vi "Measurement Logic.vi"(8 "error in":errorcluster, 9 "measurement configuration":T2 {"PAYLOAD" format="%x"; "TYPE" items=["CAN Data"=0, "CAN Remote"=1, "CAN Bus Error"=2, "CAN 2.0 Data"=8, "CAN FD Data"=16, "CAN FD+BRS Data"=24, "J1939 Data"=192, "Delay"=224, "Log Trigger"=225, "Start Trigger"=226]; "IDENTIFIER" format="%x"; "Baudrate" format="%x"; "FD Baudrate" format="%x"}, 10 "measure call context in":refnum<class "Measure Call Context.lvclass">) -> (0 "error out":errorcluster, 1 "measurement results":T1, 2 "measure call context out":refnum<class "Measure Call Context.lvclass">)   [LabVIEW 2025, in "CAN-LIN Frame Generator.lvclass"]
doc: "Contains the core logic for executing the measurement."
uses:
  CAN-LIN Frame Generator.lvclass
  <vilib>/Plug-In SDKs/Measurements/Measure Call Context/Measure Call Context.lvclass
  Measurement Configuration.ctl
  Measurement Results.ctl
  <vilib>/xnet/xnet.llb/XNET Frame CAN.ctl
  <vilib>/xnet/xnet.llb/XNET Frame Type CAN.ctl
  <vilib>/xnet/xnet.llb/XNET Create Session (Frame Output Stream).vi
  <vilib>/xnet/xnet.llb/XNET Write (Frame CAN).vi
  <vilib>/xnet/xnet.llb/XNET Wait (Transmit Complete).vi
  <extravilib>/ChannelInstances/Event Messenger-bool/Instantiate.vi
  <resource>/objmgr/xnet.rc
  session-management/xnetCAN/Session Management xnetCAN.lvlib
  <vilib>/Plug-In SDKs/Clients/Session Management V1/Session Reservation/Session Reservation.lvclass
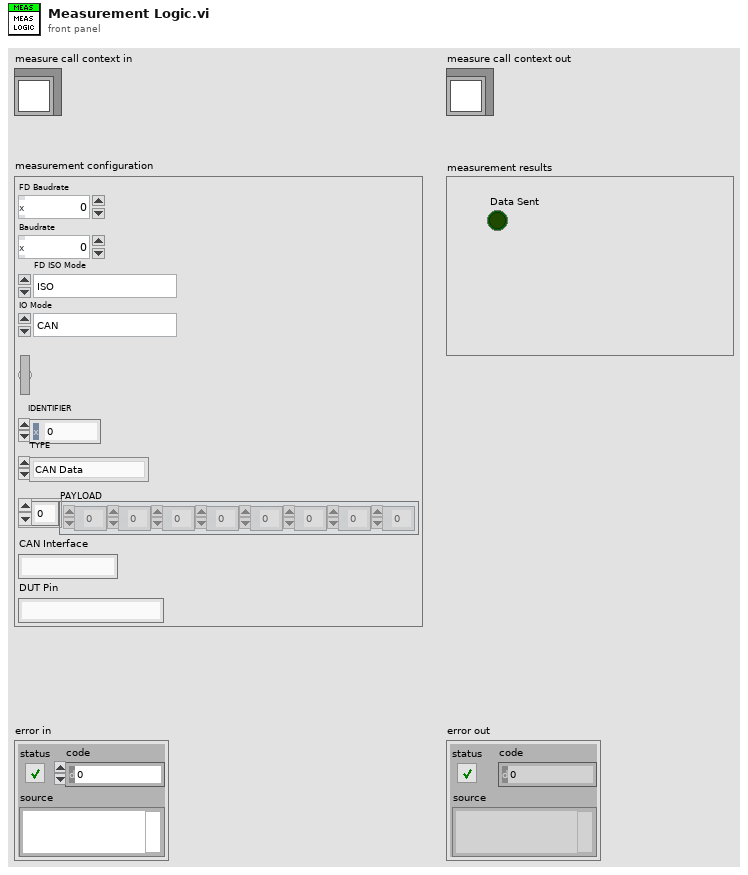
[diagram p1: front panel]
types:
  T1 = typedef "CAN-LIN Frame Generator.lvclass/Measurement Results.ctl" = cluster{"Data Sent":bool}
  T2 = typedef "CAN-LIN Frame Generator.lvclass/Measurement Configuration.ctl" = cluster{"FD Baudrate":u32, "Baudrate":u32, "FD ISO Mode":enum32{"ISO", "Legacy ISO", "Non-ISO"}, "IO Mode":enum32{"CAN", "CAN FD", "CAN FD + BRS"}, "Termination CAN":bool, "IDENTIFIER":u32, "TYPE":u32, "PAYLOAD":u32[], "CAN Interface":string, "DUT Pin":string}
  T3 = typedef "XNET Frame CAN.ctl" = cluster{"timestamp":timestamp, "payload":u8[], "identifier":u32, "type":T4, "extended?":bool, "echo?":bool}
  T4 = typedef "XNET Frame Type CAN.ctl" = u8
  T5 = typedef "Event Messenger-bool.lvlib/))Channel.ctl" = refnum<queue>
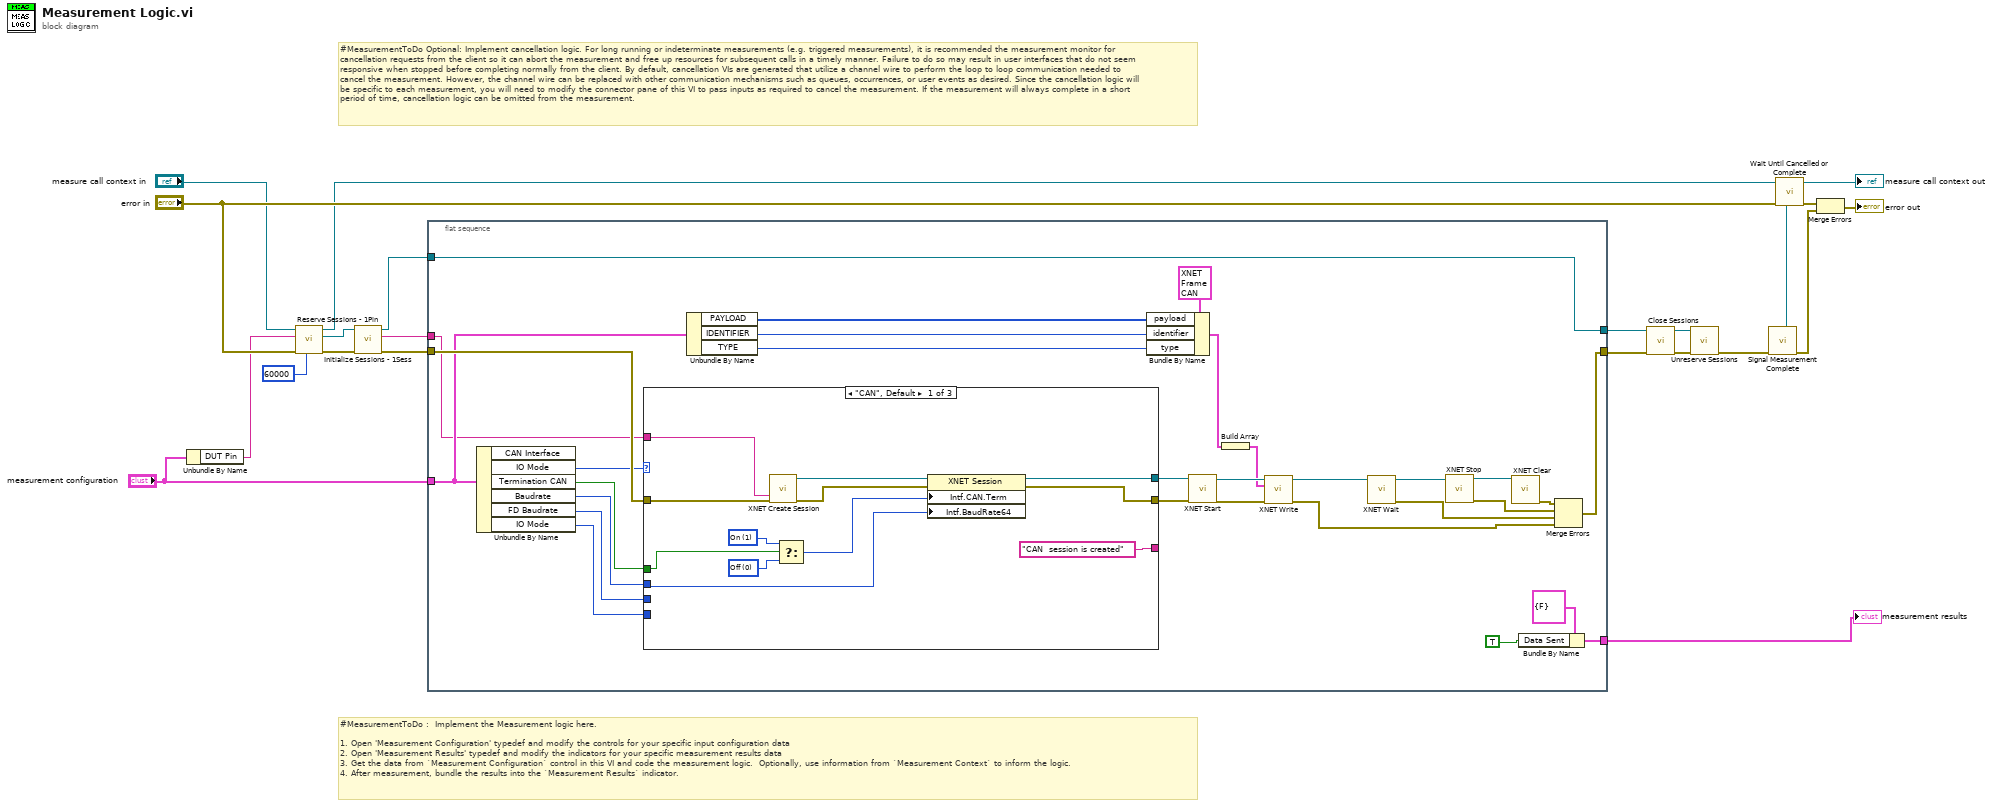
[diagram p0: block diagram]
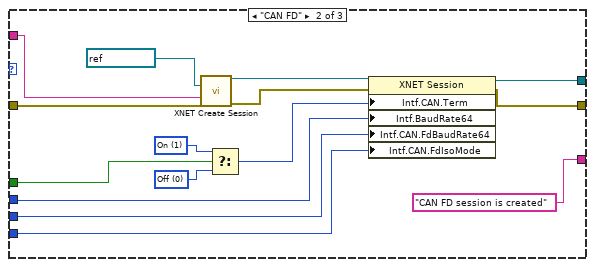
[diagram p2: hidden frame]
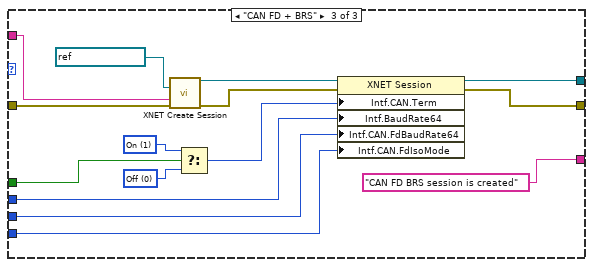
[diagram p3: hidden frame]
diagram:
  # "#MeasurementToDo Optional: Implement cancellation logic. For long running or indeterminate measurements (e.g. triggered measurements), it is recommended the measurement monitor for cancellation requests from the client so it can abort the measurement and free up resources for subsequent calls in a timely manner. Failure to do so may result in user interfaces that do not seem responsive when stopped before completing normally from the client. By default, cancellation VIs are generated that utilize a channel wire to perform the loop to loop communication needed to cancel the measurement. However, the channel wire can be replaced with other communication mechanisms such as queues, occurrences, or user events as desired. Since the cancellation logic will be specific to each measurement, you will need to modify the connector pane of this VI to pass inputs as required to cancel the measurement. If the measurement will always complete in a short period of time, cancellation logic can be omitted from the measurement."
  # "#MeasurementToDo :  Implement the Measurement logic here.\n\n1. Open 'Measurement Configuration' typedef and modify the controls for your specific input configuration data\n2. Open 'Measurement Results' typedef and modify the indicators for your specific measurement results data\n3. Get the data from `Measurement Configuration` control in this VI and code the measurement logic.  Optionally, use information from `Measurement Context` to inform the logic.\n4. After measurement, bundle the results into the `Measurement Results` indicator."
  n1 = Unbundle By Name("measurement configuration") -> ("DUT Pin"=w1:string)
  n2 = call <vilib>:"Reserve Sessions - 1Pin.vi"("timeout (ms)"=60000 ("timeout in milliseconds"), "error in"="error in", "pin or relay name"=w1, "measurement context in"="measure call context in") -> ("error out"=w11:errorcluster, "session reservation out"=w14:refnum<class "Session Reservation.lvclass">, "measurement context out"=w12:refnum<class "Measure Call Context.lvclass">)  [unwired: 5 in]
  n3 = call "Initialize Sessions - 1Sess.vi"("error in"=w11, "session reservation in"=w14) -> ("error out"=w10:errorcluster, "session"=w3:string, "session reservation out"=w4:refnum<class "Session Reservation.lvclass">)  [unwired: 6 in, 1 out]
  n4 = flat-sequence {
    tunnel: "measurement configuration" -> [w28]
    tunnel: w10 -> [w52]
    tunnel: [w30] -> w7
    tunnel: [w42] -> w17
    tunnel: [w24] -> w5
    tunnel: w4 -> [w24]
    tunnel: w3 -> [w23]
    frame #0 {
      n5 = Unbundle By Name(w28) -> ("IO Mode"=w40:enum32{"CAN", "CAN FD", "CAN FD + BRS"}, "Termination CAN"=w51:bool, "Baudrate"=w50:u32, "FD Baudrate"=w49:u32, "IO Mode"=w48:enum32{"CAN", "CAN FD", "CAN FD + BRS"})  [unwired: 1 out]
      n6 = case shown="\"CAN\", Default" w40 {
        tunnel: [w59 w69 w88] -> w47
        tunnel: w52 -> [w58 w73 w83]
        tunnel: [w57 w68 w82] -> w46
        tunnel: w51 -> [w56 w72 w87]
        tunnel: w50 -> [w55 w71 w86]
        tunnel: w49 -> [_ w67 w85]
        tunnel: w48 -> [_ w70 w84]
        tunnel: ["CAN  session is created" ("message") "CAN FD session is created" ("message") "CAN FD BRS session is created" ("message")] -> _
        tunnel: w23 -> [w53 w65 w80]
        frame "CAN", Default {
          w62 = u32 1 items=["Off", "On"] ("Interface:CAN:Termination")
          w61 = u32 0 items=["Off", "On"] ("Interface:CAN:Termination")
          n7 = call-poly <vilib>:"XNET Create Session.vi"("interface"=w53, "error in (no error)"=w58) -> ("session out"=w64:refnum<k21>, "error out"=w63:errorcluster)  [unwired: 12 in]
          n8 = Select(t=w62, s=w56, f=w61) -> (s? t:f=w60:u32)
          n9 = property class="XNET Session"(reference=w64, error in=w63, "Intf.CAN.Term"=w60, "Intf.BaudRate64"=w55) -> (reference out=w59:refnum<k21>, error out=w57:errorcluster)
        }
        frame "CAN FD" {
          w76 = u32 1 items=["Off", "On"] ("Interface:CAN:Termination")
          w75 = u32 0 items=["Off", "On"] ("Interface:CAN:Termination")
          n10 = call-poly <vilib>:"XNET Create Session.vi"("cluster (:memory:)"=refnum<k21> ":can_fd:", "interface"=w65, "error in (no error)"=w73) -> ("session out"=w78:refnum<k21>, "error out"=w77:errorcluster)  [unwired: 11 in]
          n11 = Select(t=w76, s=w72, f=w75) -> (s? t:f=w74:u32)
          n12 = property class="XNET Session"(reference=w78, error in=w77, "Intf.CAN.Term"=w74, "Intf.BaudRate64"=w71, "Intf.CAN.FdBaudRate64"=w67, "Intf.CAN.FdIsoMode"=w70) -> (reference out=w69:refnum<k21>, error out=w68:errorcluster)
        }
        frame "CAN FD + BRS" {
          w91 = u32 1 items=["Off", "On"] ("Interface:CAN:Termination")
          w90 = u32 0 items=["Off", "On"] ("Interface:CAN:Termination")
          n13 = call-poly <vilib>:"XNET Create Session.vi"("cluster (:memory:)"=refnum<k21> ":can_fd_brs:", "interface"=w80, "error in (no error)"=w83) -> ("session out"=w93:refnum<k21>, "error out"=w92:errorcluster)  [unwired: 11 in]
          n14 = Select(t=w91, s=w87, f=w90) -> (s? t:f=w89:u32)
          n15 = property class="XNET Session"(reference=w93, error in=w92, "Intf.CAN.Term"=w89, "Intf.BaudRate64"=w86, "Intf.CAN.FdBaudRate64"=w85, "Intf.CAN.FdIsoMode"=w84) -> (reference out=w88:refnum<k21>, error out=w82:errorcluster)
        }
      }
      n16 = Unbundle By Name(w28) -> ("PAYLOAD"=w27:u32[], "IDENTIFIER"=w26:u32, "TYPE"=w25:u32)
      n17 = Bundle By Name(cluster=T3 {"timestamp"=timestamp(0 s since 1904-01-01), "payload"=[1, 2, 3, 4, 5, 6, 7, 8], "identifier"=2, "type"=0, "extended?"=FALSE, "echo?"=FALSE} ("CAN frame"), "payload"=w27, "identifier"=w26, "type"=w25) -> (w38:T3)
      n18 = call <vilib>:"XNET Start.vi"("session in"=w47, "error in (no error)"=w46) -> ("session out"=w45:refnum<k21>, "error out"=w44:errorcluster)  [unwired: 12 in]
      n19 = Build Array(w38) -> (w37:T3[])
      n20 = call-poly <vilib>:"XNET Write.vi"("session in"=w45, "data"=w37, "error in (no error)"=w44) -> ("session out"=w36:refnum<k21>, "error out"=w29:errorcluster)  [unwired: 11 out]
      n21 = call-poly <vilib>:"XNET Wait.vi"("session in"=w36) -> ("session out"=w35:refnum<k21>, "error out"=w31:errorcluster)  [unwired: 13 in]
      n22 = call <vilib>:"XNET Stop.vi"("session in"=w35) -> ("session out"=w34:refnum<k21>, "error out"=w32:errorcluster)  [unwired: 13 in]
      n23 = call <vilib>:"XNET Clear.vi"("session in"=w34) -> ("error out"=w33:errorcluster)  [unwired: 14 in]
      n24 = Bundle By Name(cluster=T1 {"Data Sent"=FALSE} ("measurement results"), "Data Sent"=TRUE) -> (w42:T1)
      n25 = Merge Errors(w33, w32, w31, w29) -> (w30:errorcluster)
    }
  }
  n26 = call <vilib>:"Close Sessions.vi"("error in"=w7, "session reservation in"=w5) -> ("error out"=w9:errorcluster, "session reservation out"=w8:refnum<class "Session Reservation.lvclass">)  [unwired: 8 in]
  n27 = call <vilib>:"Unreserve Sessions.vi"("error in"=w9, "session reservation in"=w8) -> ("error out"=w6:errorcluster)  [unwired: 9 in]
  n28 = call "Signal Measurement Complete.vi"("error in (no error)"=w6) -> ("error out"=w20:errorcluster, "done channel"=w21:T5)  [unwired: 9 in]
  n29 = call "Wait Until Cancelled or Complete.vi"("done channel"=w21, "error in (no error)"="error in", "measure call context in"=w12) -> ("error out"=w19:errorcluster, "measure call context out"=→"measure call context out":refnum<class "Measure Call Context.lvclass">)  [unwired: 7 in]
  n30 = Merge Errors(w19, w20) -> (→"error out":errorcluster)
  "measurement results" <- w17
